vi "Validate_Permission.vi"(8 "error in (no error)":errorcluster, 10 "file?":bool, 11 "IB_Destination in":refnum<class "IB_Destination.lvclass">) -> (0 "error out":errorcluster, 2 "valid?":bool, 3 "IB_Destination out":refnum<class "IB_Destination.lvclass">)   [LabVIEW 2020, in "IB_Destination.lvclass"]
uses:
  <vilib>/AppBuilder/IB_Classes/Destination/IB_Destination.lvclass
  <vilib>/AppBuilder/IB_Classes/Destination/IB_Destination.lvclass/IB_Destination.ctl
  AppLibs/distkit/MDF/NI_MDF.lvlib
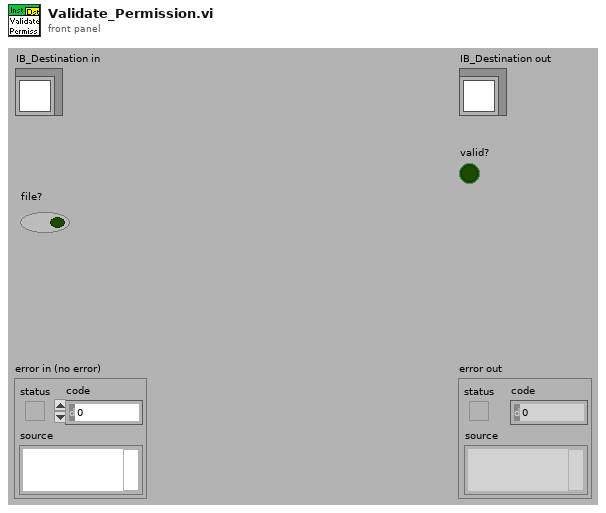
[diagram p1: front panel]
types:
  T1 = typedef "NI_MDF.lvlib/MDFBDPAddFilePathType.ctl" = i32
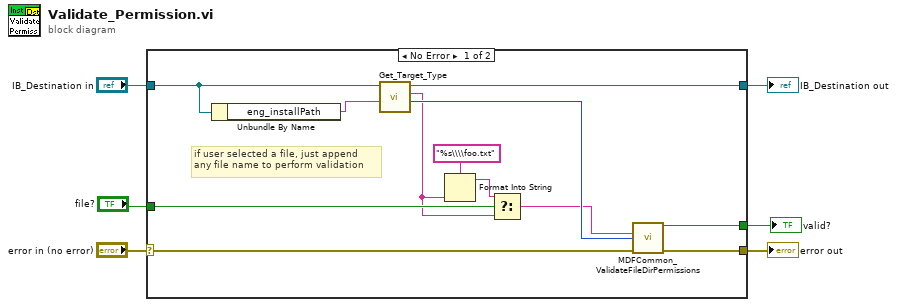
[diagram p0: block diagram]
diagram:
  n1 = case shown="No Error" "error in (no error)" {
    selector: "error in (no error)" -> [w13 w20]
    tunnel: [w12 w20] -> w5
    tunnel: [w16 w19] -> w3
    tunnel: "IB_Destination in" -> [w17 w19]
    tunnel: [w14 _] -> w2
    tunnel: "file?" -> [w11 _]
    frame No Error {
      # "if user selected a file, just append\nany file name to perform validation"
      n2 = Unbundle By Name(w17) -> ("eng_installPath"=w18:string)
      n3 = call-dynamic "Get_Target_Type.vi"("install path"=w18, "IB_Destination in"=w17) -> ("path for target type"=w15:T1, "path for target"=w8:string, "IB_Destination out"=w16:refnum<class "IB_Destination.lvclass">)  [unwired: 2 in, 5 out]
      n4 = Format Into String(format string="%s\\\\foo.txt", w8) -> (resulting string=w7:string)  [unwired: 2 in, 1 out]
      n5 = Select(t=w7, s=w11, f=w8) -> (s? t:f=w10:string)
      n6 = call "MDFCommon_ValidateFileDirPermissions.vi"("pathForTarget"=w10, "path for target type"=w15, "error in (no error)"=w13) -> ("result"=w14:bool, "error out"=w12:errorcluster)  [unwired: 11 in]
    }
    frame Error {
    }
  }
  "error out" <- w5
  "IB_Destination out" <- w3
  "valid?" <- w2
